vi "Main.vi"() -> ()   [LabVIEW 2012]
uses:
  Consumer Message.ctl
  <vilib>/ErrorRing/Error Ring.xnode
panel:
  in  "Producer Error":bool
  in  "Consumer Error":bool
  out "Consumer Shutdown?":bool
  out "State to Execute":string
  out "High Priority?":bool
  out "Backlog":u8(slide) scale=0.0..100.0
  out "Processed Value":i32
  in  "High Priority Message":bool
  in  "Normal Priority Message":bool
  in  "Stop":bool
  # "Number of enqueued\nmessages waiting to\nbe processed"
  # "Current data being\nprocessed in consumer loop"
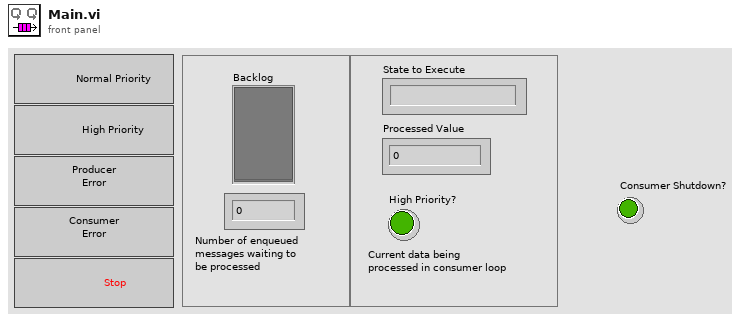
[diagram p1: front panel]
types:
  T1 = typedef "Consumer Message.ctl" = cluster{"Consumer State":string, "Boolean Data":bool, "Numeric Data":i32, "Error":errorcluster}
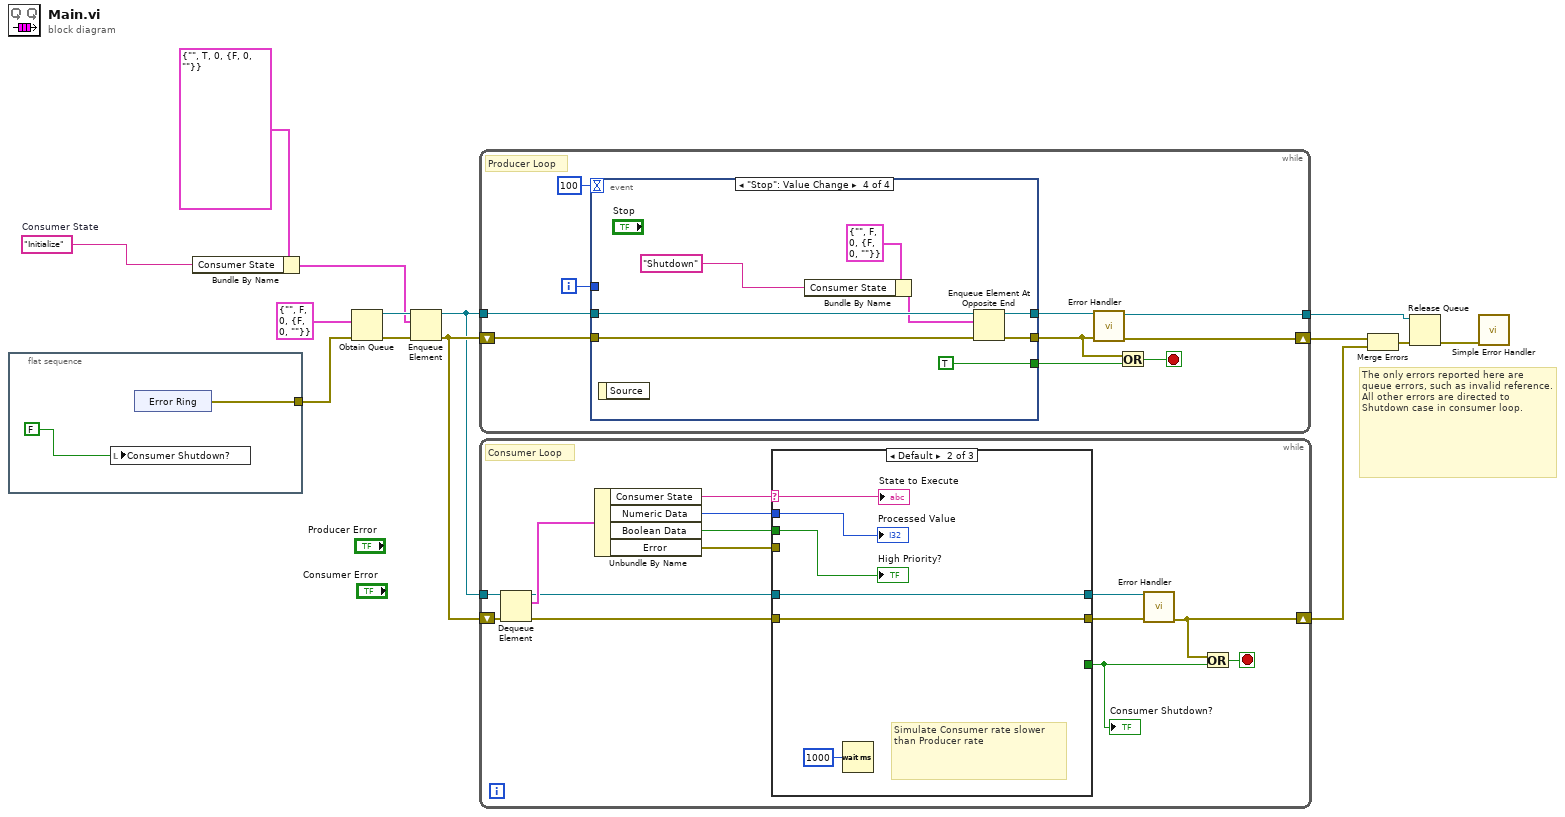
[diagram p0: block diagram]
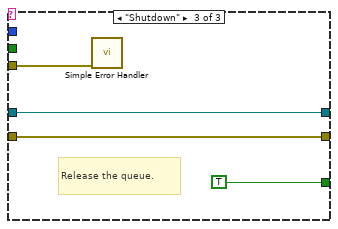
[diagram p3: hidden frame]
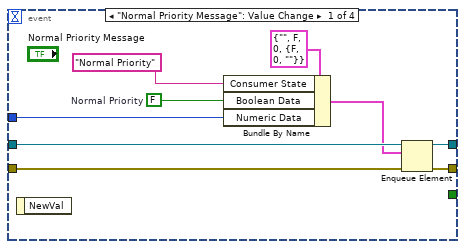
[diagram p4: hidden frame]
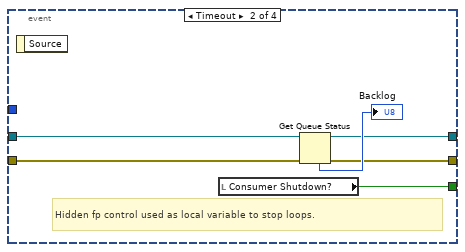
[diagram p5: hidden frame]
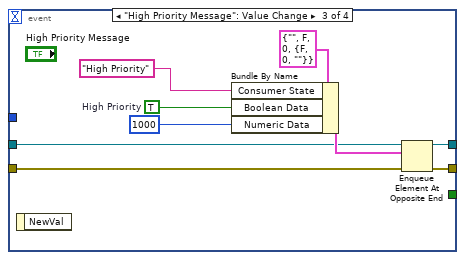
[diagram p6: hidden frame]
diagram:
  w6 = "Initialize"  # Consumer State
  # "The only errors reported here are queue errors, such as invalid reference.  All other errors are directed to Shutdown case in consumer loop."
  n1 = flat-sequence {
    tunnel: [w15] -> w9
    frame #0 {
      n2 = local write "Consumer Shutdown?"(FALSE ("Stop Loops (local)")) -> ()
      n3 = xnode "Error Ring"() -> ("error out"=w15:errorcluster)
    }
  }
  n4 = Bundle By Name(cluster=T1 {"Consumer State"="", "Boolean Data"=TRUE, "Numeric Data"=0, "Error"={"status"=FALSE, "code"=0, "source"=""}} ("Consumer Message"), "Consumer State"=w6) -> (w7:T1)
  n5 = Obtain Queue(element data type=T1 {"Consumer State"="", "Boolean Data"=FALSE, "Numeric Data"=0, "Error"={"status"=FALSE, "code"=0, "source"=""}}, error in (no error)=w9) -> (queue out=w11:refnum<queue>, error out=w14:errorcluster)  [unwired: 3 in, 1 out]
  n6 = Enqueue Element(queue=w11, element=w7, error in (no error)=w14) -> (queue out=w10:refnum<queue>, error out=w12:errorcluster)  [unwired: 1 in, 1 out]
  n7 = while {
    tunnel: w10 -> [w27]
    shift-right: [w19] -> w4
    shift-left: w12 -> [w26]
    tunnel: [w18] -> w1
    i -> [w25]
    stop <- w21 stop-if-true
    # "Producer Loop"
    n8 = event shown="[3] \"Stop\": Value Change" {
      selector: _ -> [_ _ _ _]
      dyn-events: _ -> [_ _ _ _]
      timeout: 100 -> [_ _ _ _]
      tunnel: w27 -> [w36 w40 w43 w59]
      tunnel: w26 -> [w34 w39 w50 w57]
      tunnel: [w35 w38 w51 w56] -> w20
      tunnel: [_ w42 _ TRUE] -> w22
      tunnel: w25 -> [w33 _ _ _]
      tunnel: [w29 w37 w46 w55] -> w24
      event "Normal Priority Message": Value Change {
        w30 = FALSE  # Normal Priority
        n9 = event-data() -> ()  [unwired: 1 in, 1 out]
        n10 = Bundle By Name(cluster=T1 {"Consumer State"="", "Boolean Data"=FALSE, "Numeric Data"=0, "Error"={"status"=FALSE, "code"=0, "source"=""}}, "Consumer State"="Normal Priority" ("String Data"), "Boolean Data"=w30, "Numeric Data"=w33) -> (w32:T1)
        n11 = Enqueue Element(queue=w36, element=w32, error in (no error)=w34) -> (queue out=w29:refnum<queue>, error out=w35:errorcluster)  [unwired: 1 in, 1 out]
      }
      event Timeout {
        # "Hidden fp control used as local variable to stop loops."
        n12 = event-data() -> ()  [unwired: 1 in, 1 out]
        n13 = local read "Consumer Shutdown?"() -> (w42:bool)
        n14 = Get Queue Status(queue=w40, error in (no error)=w39) -> (queue out=w37:refnum<queue>, error out=w38:errorcluster, # elements in queue=→"Backlog":i32)  [unwired: 1 in, 5 out]
      }
      event "High Priority Message": Value Change {
        w45 = TRUE  # High Priority
        n15 = event-data() -> ()  [unwired: 1 in, 1 out]
        n16 = Bundle By Name(cluster=T1 {"Consumer State"="", "Boolean Data"=FALSE, "Numeric Data"=0, "Error"={"status"=FALSE, "code"=0, "source"=""}}, "Consumer State"="High Priority" ("String Data"), "Boolean Data"=w45, "Numeric Data"=1000) -> (w48:T1)
        n17 = Enqueue Element At Opposite End(queue=w43, element=w48, error in (no error)=w50) -> (queue out=w46:refnum<queue>, error out=w51:errorcluster)  [unwired: 1 in, 1 out]
      }
      event "Stop": Value Change {
        n18 = event-data() -> ()  [unwired: 1 in, 1 out]
        n19 = Bundle By Name(cluster=T1 {"Consumer State"="", "Boolean Data"=FALSE, "Numeric Data"=0, "Error"={"status"=FALSE, "code"=0, "source"=""}}, "Consumer State"="Shutdown") -> (w52:T1)
        n20 = Enqueue Element At Opposite End(queue=w59, element=w52, error in (no error)=w57) -> (queue out=w55:refnum<queue>, error out=w56:errorcluster)  [unwired: 1 in, 1 out]
      }
    }
    n21 = call "Error Handler.vi"("error in"=w20, "queue in"=w24) -> ("error out"=w19:errorcluster, "queue out"=w18:refnum<queue>)  [unwired: 8 in]
    n22 = Or(x=w20, y=w22) -> (x .or. y?=w21:bool)
  }
  n23 = while {
    tunnel: w10 -> [w73]
    shift-right: [w62] -> w5
    shift-left: w12 -> [w72]
    stop <- w63 stop-if-true
    # "Consumer Loop"
    n24 = Dequeue Element(queue=w73, error in (no error)=w72) -> (queue out=w61:refnum<queue>, element=w71:T1, error out=w60:errorcluster)  [unwired: 1 in, 1 out]
    n25 = Unbundle By Name(w71) -> ("Consumer State"=w70:string, "Numeric Data"=w69:i32, "Boolean Data"=w68:bool, "Error"=w65:errorcluster)
    n26 = case shown="Default" w70 {
      selector: w70 -> [_ w78 _]
      tunnel: [_ _ TRUE] -> w64
      tunnel: w60 -> [w74 w76 w82]
      tunnel: [w74 w76 w82] -> w67
      tunnel: w69 -> [_ w81 _]
      tunnel: w68 -> [_ w80 _]
      tunnel: w61 -> [w75 w79 w83]
      tunnel: [w75 w79 w83] -> w66
      tunnel: w65 -> [_ _ w84]
      frame "Initialize" {
      }
      frame Default {
        # "Simulate Consumer rate slower than Producer rate"
        n27 = Wait (ms)(milliseconds to wait=u32 1000) -> ()  [unwired: 1 out]
        "Processed Value" <- w81
        "High Priority?" <- w80
        "State to Execute" <- w78
      }
      frame "Shutdown" {
        # "Release the queue."
        n28 = call <vilib>:"Simple Error Handler.vi"("error in (no error)"=w84) -> ()  [unwired: 4 in, 5 out]
      }
    }
    "Consumer Shutdown?" <- w64
    n29 = call "Error Handler.vi"("error in"=w67, "queue in"=w66) -> ("error out"=w62:errorcluster)  [unwired: 8 in, 1 out]
    n30 = Or(x=w62, y=w64) -> (x .or. y?=w63:bool)
  }
  n31 = Merge Errors(w4, w5) -> (w3:errorcluster)
  n32 = Release Queue(queue=w1, error in (no error)=w3) -> (error out=w2:errorcluster)  [unwired: 1 in, 2 out]
  n33 = call <vilib>:"Simple Error Handler.vi"("error in (no error)"=w2) -> ()  [unwired: 4 in, 5 out]
